vi "the best.vi"() -> ()   [LabVIEW 2010]
panel:
  in  "Finish":bool
  # "Hardware Platform"
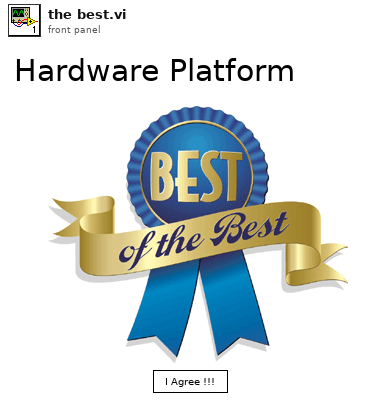
[diagram p1: front panel]
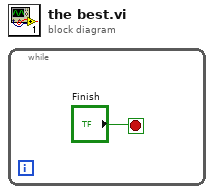
[diagram p0: block diagram]
diagram:
  n1 = while {
    stop <- "Finish" stop-if-true
  }
